vi "SUB-Make_File_Name.vi"(8 "error in (no error)":errorcluster) -> (0 "error out":errorcluster, 3 "Error(T)":bool)   [LabVIEW 2012]
panel:
  in  "Serial Nuber For Debug":string[](array[string])
  in  "Debug(T)":bool
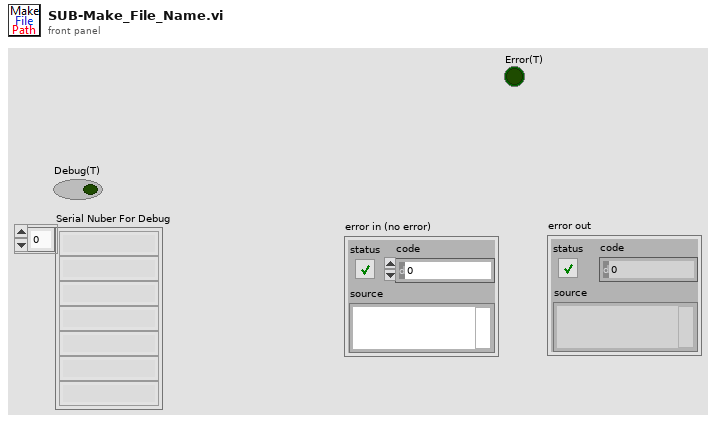
[diagram p1: front panel]
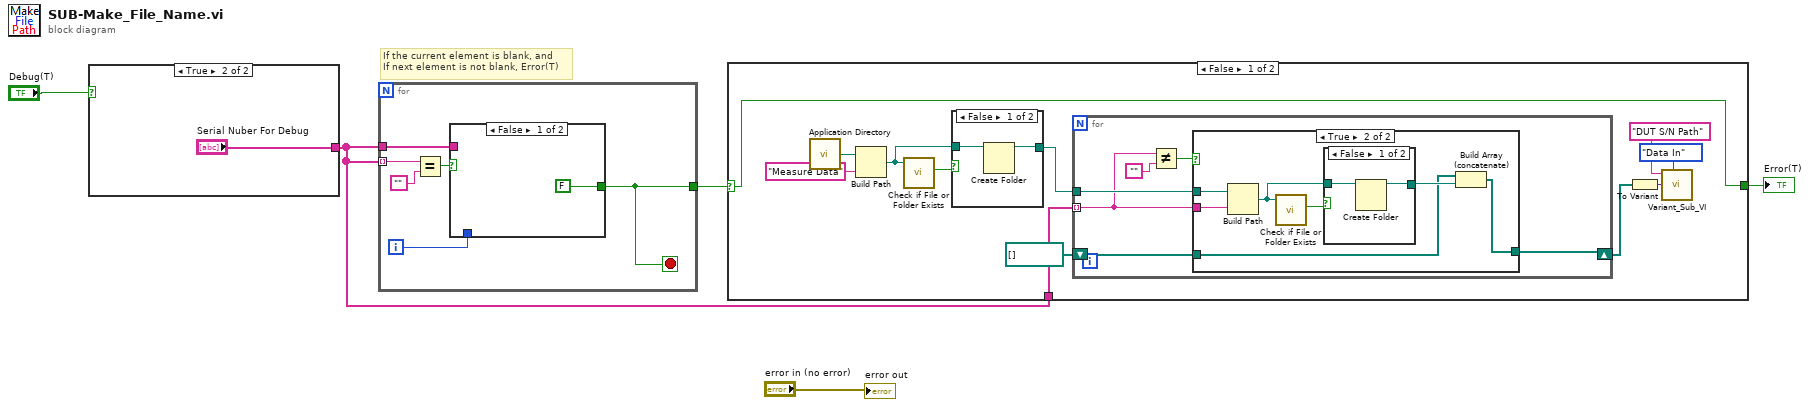
[diagram p0: block diagram]
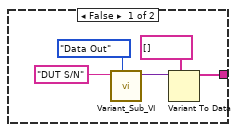
[diagram p2: hidden frame]
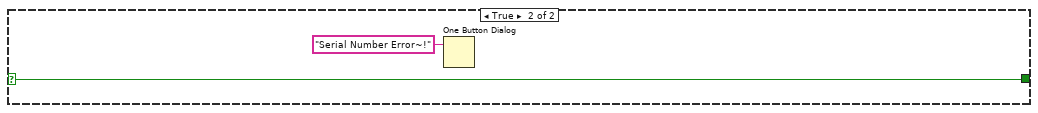
[diagram p6: hidden frame]
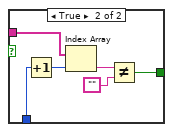
[diagram p7: hidden frame]
diagram:
  # "If the current element is blank, and \nIf next element is not blank, Error(T)"
  n1 = case shown="True" "Debug(T)" {
    tunnel: [w6 "Serial Nuber For Debug"] -> w4
    frame False {
      n2 = call "Variant_Sub_VI.vi"("Mode"=enum16{"Init", "Data In", "Data Out"}."Data Out", "Data Name"="DUT S/N") -> ("Out"=w10:variant)  [unwired: 8 in, 1 out]
      n3 = Variant To Data(type=string[] [], Variant=w10) -> (data=w6:string[])  [unwired: 1 in, 1 out]
    }
    frame True {
    }
  }
  n4 = for {
    tunnel: w4 -> [w17] mode=indexing
    tunnel: w4 -> [w14]
    tunnel: [w12] -> w5
    i -> [w13]
    stop <- w12 stop-if-true
    n5 = Equal?(x=w17, y="") -> (x = y?=w15:bool)
    n6 = case shown="False" w15 {
      tunnel: w14 -> [_ w24]
      tunnel: w13 -> [_ w23]
      tunnel: [FALSE w19] -> w12
      frame False {
      }
      frame True {
        n7 = Increment(x=w23) -> (x+1=w22:i32)
        n8 = Index Array(array=w24, index=w22) -> (element=w21:string)
        n9 = Not Equal?(x=w21, y="") -> (x != y?=w19:bool)
      }
    }
  }
  n10 = case shown="False" w5 {
    selector: w5 -> [w27 w57]
    tunnel: w4 -> [w28 _]
    tunnel: [w27 w57] -> w3
    frame False {
      n11 = call <vilib>:"Application Directory.vi"() -> ("Application Directory"=w32:path)
      n12 = Build Path(base path=w32, name or relative path="Measure Data") -> (appended path=w29:path)
      n13 = call <vilib>:"Check if File or Folder Exists.vi"("path"=w29) -> ("file or folder exists?"=w30:bool)  [unwired: 8 in, 2 out]
      n14 = case shown="False" w30 {
        tunnel: w29 -> [w55 w56]
        tunnel: [w54 w56] -> w36
        frame False {
          n15 = Create Folder(path (use dialog)=w55) -> (created path=w54:path)  [unwired: 2 in, 2 out]
        }
        frame True {
        }
      }
      n16 = for {
        tunnel: w36 -> [w42]
        tunnel: w28 -> [w39] mode=indexing
        shift-right: [w38] -> w25
        shift-left: path[] [] -> [w37]
        n17 = Not Equal?(x=w39, y="") -> (x != y?=w40:bool)
        n18 = case shown="True" w40 {
          tunnel: w42 -> [_ w48]
          tunnel: w39 -> [_ w47]
          tunnel: [w43 w45] -> w38
          tunnel: w37 -> [w43 w44]
          frame False {
          }
          frame True {
            n19 = Build Path(base path=w48, name or relative path=w47) -> (appended path=w49:path)
            n20 = call <vilib>:"Check if File or Folder Exists.vi"("path"=w49) -> ("file or folder exists?"=w50:bool)  [unwired: 8 in, 2 out]
            n21 = case shown="False" w50 {
              tunnel: w49 -> [w52 w53]
              tunnel: [w51 w53] -> w46
              frame False {
                n22 = Create Folder(path (use dialog)=w52) -> (created path=w51:path)  [unwired: 2 in, 2 out]
              }
              frame True {
              }
            }
            n23 = Build Array (concatenate)(w44, w46) -> (w45:path[])
          }
        }
      }
      n24 = To Variant(anything=w25) -> (Variant=w33:variant)
      n25 = call "Variant_Sub_VI.vi"("Mode"=enum16{"Init", "Data In", "Data Out"}."Data In", "IN"=w33, "Data Name"="DUT S/N Path") -> ()  [unwired: 7 in, 2 out]
    }
    frame True {
      n26 = One Button Dialog(message="Serial Number Error~!") -> ()  [unwired: 1 in, 1 out]
    }
  }
  "Error(T)" <- w3
  "error out" <- "error in (no error)"
